vi "S2C_FORNAX_Proc_ExtractMsg.vi"(8 "Error In":errorcluster, 11 "DDS Message":string) -> (0 "Error Out":errorcluster, 2 "Found?":bool, 3 "VIPER Message":string)   [LabVIEW 2015]
doc: "Extracts the Viper message from the DDS data stream."
uses:
  <vilib>/regexp/Match Regular Expression.xnode
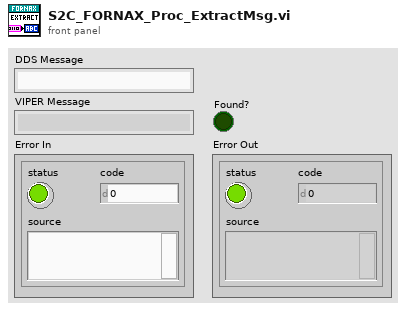
[diagram p1: front panel]
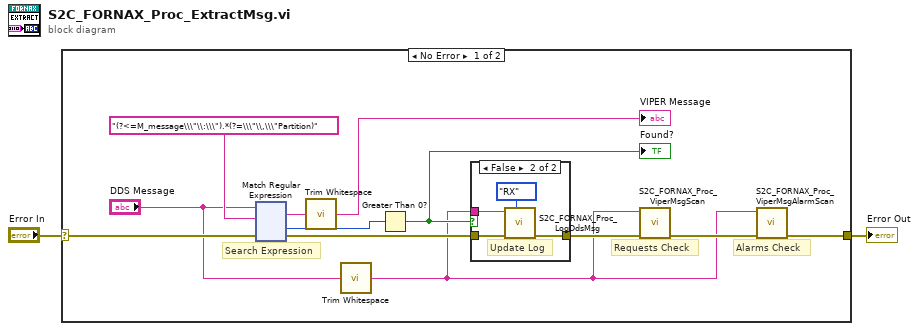
[diagram p0: block diagram]
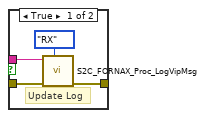
[diagram p2: hidden frame]
diagram:
  n1 = case shown="No Error" "Error In" {
    selector: "Error In" -> [w11 w134]
    tunnel: [w5 w134] -> w1
    frame No Error {
      # "Alarms Check"
      # "Requests Check"
      # "Search Expression"
      n2 = xnode "Match Regular Expression"("input string"="DDS Message", "regular expression"="(?<=M_message\\\"\\:\\\").*(?=\\\"\\,\\\"Partition)" ("format string"), "error in"=w11) -> ("whole match"=w13:string, "offset past match"=w12:i32, "error out"=w10:errorcluster)  [unwired: 3 in, 2 out]
      n3 = call <vilib>:"Trim Whitespace.vi"("string"=w13) -> ("trimmed string"=→"VIPER Message":string)  [unwired: 1 in]
      n4 = call <vilib>:"Trim Whitespace.vi"("string"="DDS Message") -> ("trimmed string"=w3:string)  [unwired: 1 in]
      n5 = Greater Than 0?(x=w12) -> (x > 0?=w7:bool)
      "Found?" <- w7
      n6 = case shown="False" w7 {
        tunnel: w10 -> [w18 w22]
        tunnel: [w17 w21] -> w9
        tunnel: w3 -> [w15 w19]
        frame True {
          # "Update Log"
          n7 = call "S2C_FORNAX_Proc_LogVipMsg.vi"("Direction"=enum16{"TX", "RX"}."RX", "Error In"=w18, "Msg In"=w15) -> ("Error Out"=w17:errorcluster)  [unwired: 7 in, 1 out]
        }
        frame False {
          # "Update Log"
          n8 = call "S2C_FORNAX_Proc_LogDdsMsg.vi"("Direction"=enum16{"TX", "RX"}."RX", "Error In"=w22, "Msg In"=w19) -> ("Error Out"=w21:errorcluster)  [unwired: 7 in, 1 out]
        }
      }
      n9 = call "S2C_FORNAX_Proc_ViperMsgScan.vi"("Error In"=w9, "Message"=w3) -> ("Error Out"=w6:errorcluster)  [unwired: 9 in]
      n10 = call "S2C_FORNAX_Proc_ViperMsgAlarmScan.vi"("Error In"=w6, "Message"=w3) -> ("Error Out"=w5:errorcluster)  [unwired: 9 in]
    }
    frame Error {
    }
  }
  "Error Out" <- w1
